vi "DMR_GetImageRequestBufferImageData.vi"(0 "driver handle IN":u32, 1 "request number IN":u32, 2 "bytes per pixel IN":u32, 4 "X-offset IN":u32, 5 "Y-offset IN":u32, 7 "height IN":u32, 9 "width IN":u32) -> (14 "driver handle OUT":u32, 15 "request number OUT":u32, 17 "image OUT":u32[][](array[numeric]), 19 "error code OUT":i32)   [LabVIEW 2016]
doc: "Returns an AOI of raw image data belonging to the specified request.\n\nThe 'request number IN' parameter can be obtained from the DMR_ImageRequestWaitFor VI.\n\nPlease note, that the usage of the sub-VIs called by this VI (e.g. 'DMR_GetImageRequestBufferImageData8Bit') perform much more efficient as no data conversion has to be performed within LabVIEW. For applications with known pixel formats therefore these VIs should be used.\n\nSee also:\nDMR_GetImageRequestBufferChannelData\n\nThe 'error code OUT' terminal will deliver 0 if successful or a negative error code otherwise. A list of valid error codes and their meaning can be found in the manual about this interface."
panel:
  # "OUTPUT"
  # "INPUT"
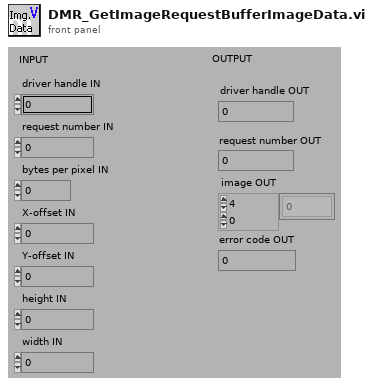
[diagram p1: front panel]
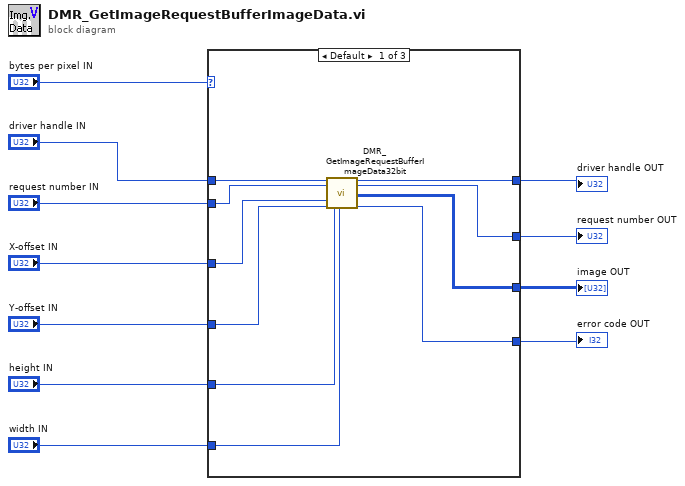
[diagram p0: block diagram]
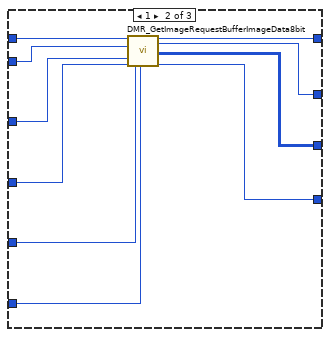
[diagram p2: hidden frame]
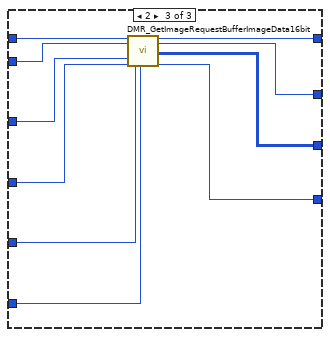
[diagram p3: hidden frame]
diagram:
  n1 = case shown="Default" "bytes per pixel IN" {
    tunnel: "driver handle IN" -> [w21 w31 w41]
    tunnel: "request number IN" -> [w20 w30 w40]
    tunnel: "X-offset IN" -> [w19 w29 w39]
    tunnel: "Y-offset IN" -> [w18 w28 w38]
    tunnel: "height IN" -> [w17 w27 w37]
    tunnel: [w15 w26 w35] -> w5
    tunnel: [w12 w25 w32] -> w4
    tunnel: "width IN" -> [w16 w24 w36]
    tunnel: [w14 w23 w34] -> w2
    tunnel: [w13 w22 w33] -> w1
    frame Default {
      n2 = call "DMR_GetImageRequestBufferImageData32bit.vi"("driver handle IN"=w21, "request number IN"=w20, "X-offset"=w19, "Y-offset"=w18, "height"=w17, "width"=w16) -> ("driver handle OUT"=w15:u32, "request number OUT"=w14:u32, "image OUT"=w13:u32[][], "error code OUT"=w12:i32)  [unwired: 10 in]
    }
    frame 1 {
      n3 = call "DMR_GetImageRequestBufferImageData8bit.vi"("driver handle IN"=w31, "request number IN"=w30, "X-offset"=w29, "Y-offset"=w28, "height"=w27, "width"=w24) -> ("driver handle OUT"=w26:u32, "request number OUT"=w23:u32, "image OUT"=w22:u8[][], "error code OUT"=w25:i32)  [unwired: 10 in]
    }
    frame 2 {
      n4 = call "DMR_GetImageRequestBufferImageData16bit.vi"("driver handle IN"=w41, "request number IN"=w40, "X-offset"=w39, "Y-offset"=w38, "height"=w37, "width"=w36) -> ("driver handle OUT"=w35:u32, "request number OUT"=w34:u32, "image OUT"=w33:u16[][], "error code OUT"=w32:i32)  [unwired: 10 in]
    }
  }
  "error code OUT" <- w4
  "request number OUT" <- w2
  "image OUT" <- w1
  "driver handle OUT" <- w5
